vi "Globals.vi"() -> ()   [LabVIEW 2017, in "nifxpmath_Interpret.xnode"]
uses:
  <vilib>/rvi/FXPMathLib/FxpInterpret/XNode/nifxpmath_Interpret.xnode
panel:
  out "SmallIcon":picture
  out "NormalBanner":picture
  in  "Term Output Name":string="y"
  in  "Term Input Name":string="x"
  in  "Menu Icon ID":string="MENU_SMLBIGICON"
  in  "Term Output ID":string="TERM_Output"
  in  "Term Input ID":string="TERM_Input"
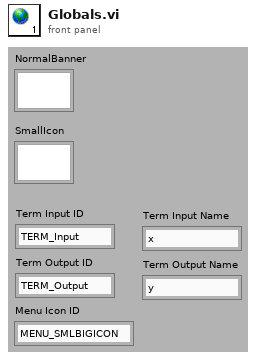
[diagram p1: front panel]
diagram:
